vi "Main Editor UI.vi"() -> ()   [LabVIEW 2013, in "Shared Memory editor node.lvclass"]
doc: "This is the main view for configuration the behavior of a module in the DCAF standard editor."
uses:
  Shared Memory editor node.lvclass
  <vilib>/NI/Configuration Framework/Controls/EventCluster.ctl
  <vilib>/NI/Configuration Framework/NISE_CEF_TreeControl.lvlib
  <vilib>/NI/Configuration Framework/Node/UserEventRef.ctl
  <vilib>/NI/Configuration Framework/Node/NISE_CEF_Node.lvclass
  <vilib>/NI/Tools/Keyed Array/KeyedArray.ctl
  <vilib>/NI/Tools/Keyed Array/Tools_KeyedArray.lvlib
  <vilib>/NI/AMC/Message.ctl
  <vilib>/NI/AMC/AMC.lvlib
  <vilib>/NI/AMC/Message Queue.ctl
  <vilib>/NI/Tag Bus/tag/tag descriptor.lvclass
  <vilib>/NI/Tag Bus Module Framework/channel/TBM channel.lvclass
  <vilib>/NI/DCAF/Tag Editor Core/Table API/Available Tag Menu/channel action event.ctl
  <vilib>/NI/DCAF/Tag Editor Core/Table API/Table Manager.lvlib
  <vilib>/NI/Configuration Framework/Node/NodeRef.ctl
  <vilib>/NI/Configuration Framework/Node/NodeChangeEvent.ctl
  <vilib>/NI/Configuration Framework/Node/CacheState.ctl
  <vilib>/NI/Configuration Framework/Node/RefreshUIEvent.ctl
  <vilib>/NI/Configuration Framework/Node/StopEvent.ctl
  <vilib>/NI/DCAF/Tag Editor Core/Table API/Table Manager/references.ctl
  <vilib>/NI/DCAF/Tag Editor Core/Table API/Table Manager/Table Manager.lvclass
  <vilib>/NI/DCAF/Tag Editor Core/Table API/Listbox/Multi Column Listbox.lvclass
  <vilib>/Utility/miscctls.llb/LVPositionTypeDef.ctl
  <vilib>/NI/DCAF UI Toolkit/Controls/DCAF UI Elements.lvlib
  <vilib>/NI/DCAF/Tag Editor Core/Table API/Table Manager/Call Back Ref Type Def.ctl
  <vilib>/NI/DCAF/Tag Editor Core/Table API/Available Tag Menu/dialog output action.ctl
  <vilib>/NI/DCAF/Tag Editor Core/Configuration Editor/Classes/Engine Parent/Engine Parent Editor Node.lvclass
  <vilib>/NI/DCAF/Tag Editor Core/Configuration Editor/Classes/Module editor node/module editor node.lvclass
  module/configuration/Shared Memory configuration.lvclass
  <vilib>/NI/Tag Bus/tag/Data Type.ctl
  Permissions Enum.ctl
  sync/sync item.ctl
  sync/sync mechanism.ctl
  <vilib>/NI/DCAF UI Toolkit/Controls/Add.ctl
  <vilib>/NI/DCAF UI Toolkit/Controls/Remove.ctl
  <vilib>/NI/DCAF UI Toolkit/Controls/Configure.ctl
panel:
  in  "user event out":refnum<user-event>
  in  "Permissions":T1=enum."Read from Memory"
  in  "data type":T2
  in  "node change":T3
  in  "cache state":T4
  in  "refresh UI":T5
  in  "stop event":T6
  in  "Tab Control":T7(tab)
  in  "Remove Button":T8
  in  "Add Button":T9
  in  "Table":i32(listbox)
  in  "settings":T10
  in  "output file string":string caption="output file string (optional)"
  in  "input file string":string caption="input file string (optional)"
  in  "minor":dbl
  in  "major":dbl
  in  "C header":bool
  in  "c header file string":string caption="C header file string (optional)"
  in  "c header file directory":path caption="C header file directory"
  in  "Shared memory name":string="dcaf_sync"
  out "Struct prototype":string="struct dcaf_sync{\n   semt_t start_sem;\n};"
  in  "sync end of cycle":T11[](array[typedef])=[{"mechanism"=enum."Semaphore", "name"=""}]
  in  "sync start of cycle":T11[](array[typedef])
  in  "Struct name":string="dcaf_sync"
  in  "Timeout (us)":i32 step=25
  in  "Enable sync":bool
  in  "user event":T13
  in  "main queue":T14
  in  "node ref":T15
  # "Shared Memory Files (<EngineName>_<\"input/output\">_<DataType>_<FileString>)"
  # "The data file names will follow a fixed format with an optional appended user file name string. File input and output classification is from the perspective of an  external process (or application) which will access the file.\n\nExample: A C application running in parallel to the DCAF based LabVIEW Real-Time EXE application will view any file that it writes to as an \"output\" data file in Linux shared memory."
  # "C Header File Generation"
  # "Generate a C header file in a \"C header file directory\" which contains shared memory mapping information for use in C applications. The default C header file name will use the configuration file name and add optional user \"C header file string\" text: \n\n<ConfigurationFileName>_<FileString>.h\n\nThe user will override the file name format if the \".h\" file extension is included. The \"version\" will be added to the header file as a #define declaration in the header file."
  # "version"
  # "Start of cycle"
  # "End of cycle (optional response)"
  # "Mechanism"
  # "Name in struct"
  # "Mechanism"
  # "Name in struct"
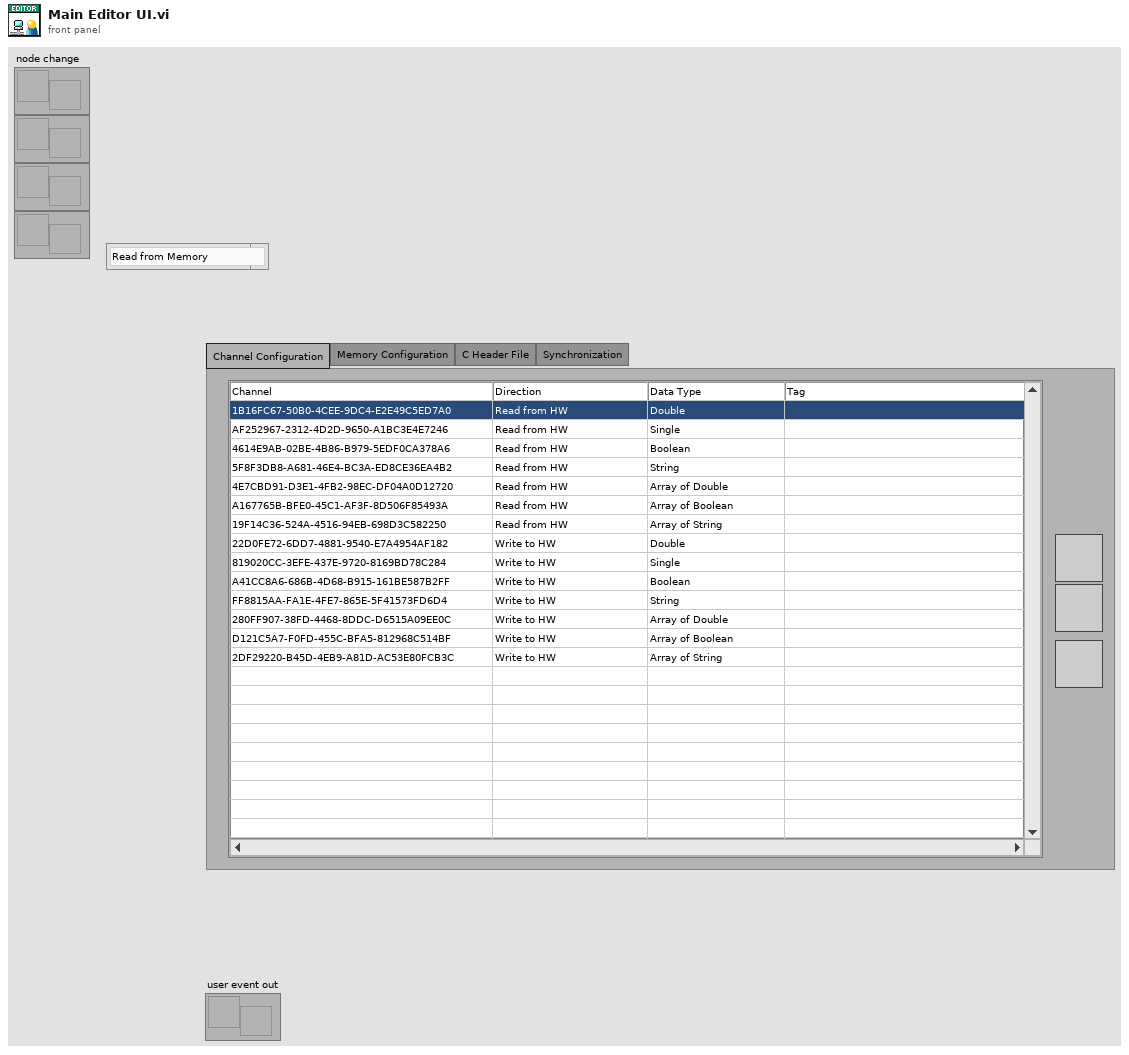
[diagram p1: front panel]
types:
  T1 = typedef "Shared Memory editor node.lvclass/Permissions Enum.ctl" = enum16{"Write to Memory", "Read from Memory"}
  T2 = typedef "tag bus.lvlib/tag descriptor.lvclass/Data Type.ctl" = enum16{"Double", "Single", "I64", "I32", "I16", "I8", "U64", "U32", "U16", "U8", "Boolean", "String", "Array of Double", "Array of Single", "Array of I64", "Array of I32", "Array of I16", "Array of I8", "Array of U64", "Array of U32", "Array of U16", "Array of U8", "Array of Boolean", "Array of String"}
  T3 = typedef "NISE_CEF_Node.lvclass/NodeChangeEvent.ctl" = refnum<user-event>
  T4 = typedef "NISE_CEF_Node.lvclass/CacheState.ctl" = refnum<user-event>
  T5 = typedef "NISE_CEF_Node.lvclass/RefreshUIEvent.ctl" = refnum<user-event>
  T6 = typedef "NISE_CEF_Node.lvclass/StopEvent.ctl" = refnum<user-event>
  T7 = enum32{"Channel Configuration", "Memory Configuration", "C Header File", "Synchronization"}
  T8 = typedef "DCAF UI Elements.lvlib/Remove.ctl" = bool
  T9 = typedef "DCAF UI Elements.lvlib/Add.ctl" = bool
  T10 = typedef "DCAF UI Elements.lvlib/Configure.ctl" = bool
  T11 = typedef "Shared Memory configuration.lvclass/sync item.ctl" = cluster{"mechanism":T12, "name":string}
  T12 = typedef "Shared Memory configuration.lvclass/sync mechanism.ctl" = enum16{"Semaphore", "Conditional Variable"}
  T13 = typedef "NISE_CEF_Node.lvclass/UserEventRef.ctl" = refnum<user-event>
  T14 = typedef "AMC.lvlib/Message Queue.ctl" = refnum<queue>
  T15 = typedef "NISE_CEF_Node.lvclass/NodeRef.ctl" = refnum<data-value>
  T16 = typedef "Table Manager.lvlib/Table Manager.lvclass/references.ctl" = cluster{"stop event":T6, "refresh UI":T5, "cache state":T4, "node change":T3, "user event out":refnum<user-event>, "main queue":T14, "user event":T13}
  T17 = typedef "LVPositionTypeDef.ctl" = cluster{"Left":i32, "Top":i32}
  T18 = typedef "Table Manager.lvlib/Table Manager.lvclass/object ref.ctl" = cluster{"engine":refnum<data-value>, "Node Ref":refnum<data-value>}
  T19 = typedef "Table Manager.lvlib/Column.lvclass/Column Descriptor.ctl" = cluster{"name":string, "caption":string, "Column Type":T20, "Params":string, "AutoSizeMode":i32, "FillWeight":sgl, "MinWidth":u32, "tooltip":string, "Enum Reference":refnum<vi>, "Channel suffix":string, "Read Only":bool, "Call Back VI":T21, "DT Dependency":i32, "name dependency":i32, "data type":T2, "Custom Column":refnum<class "Column.lvclass">}
  T20 = typedef "Table Manager.lvlib/Column.lvclass/Column Type.ctl" = enum16{"String", "Mapping", "Enum", "Custom"}
  T21 = typedef "Table Manager.lvlib/Table Manager.lvclass/Call Back Ref Type Def.ctl" = refnum<vi>
  T22 = typedef "Table Manager.lvlib/Table Manager.lvclass/Table Events.ctl" = cluster{"Menu Selection":refnum<user-event>}
  T23 = enum8{"Enabled", "Disabled", "Disabled and Grayed Out"}
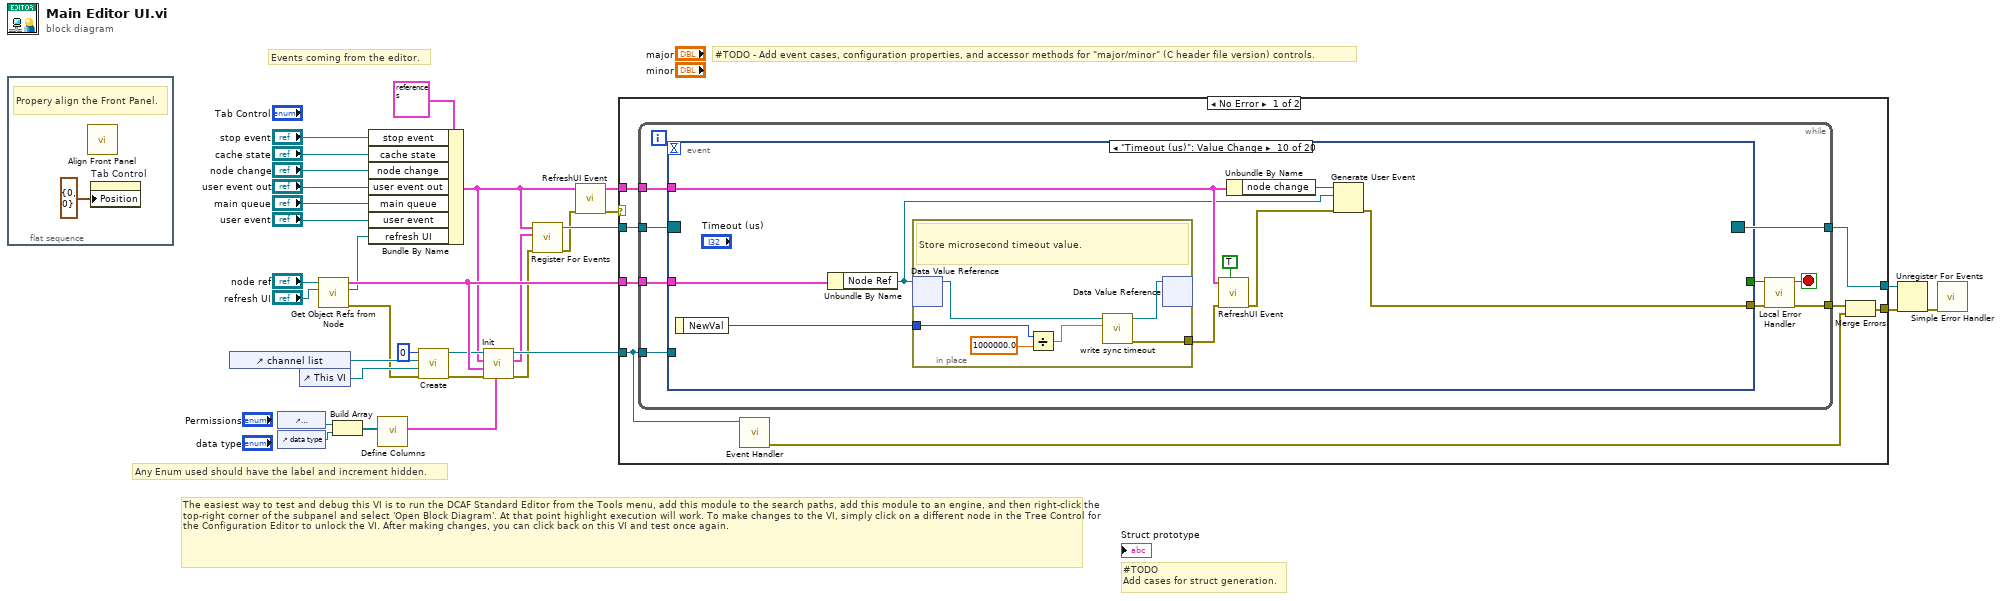
[diagram p0: block diagram]
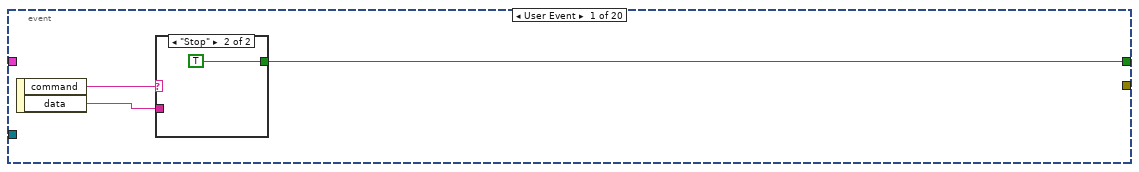
[diagram p2: hidden frame]
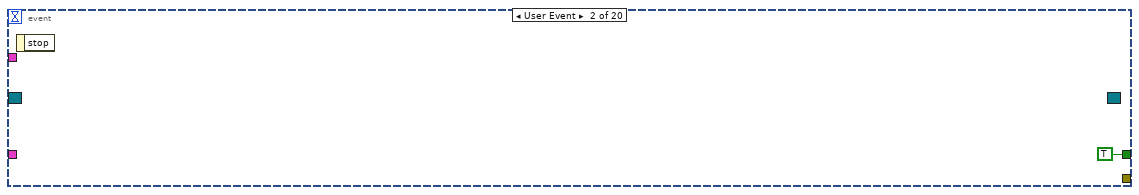
[diagram p4: hidden frame]
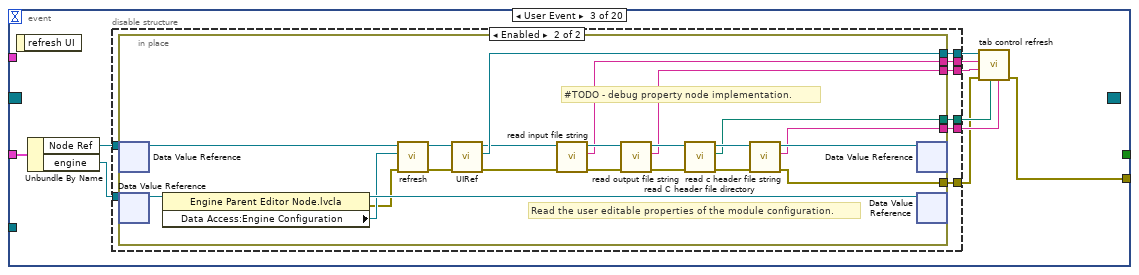
[diagram p5: hidden frame]
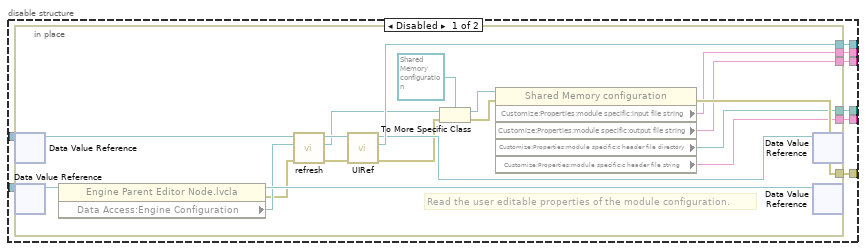
[diagram p6: hidden frame]
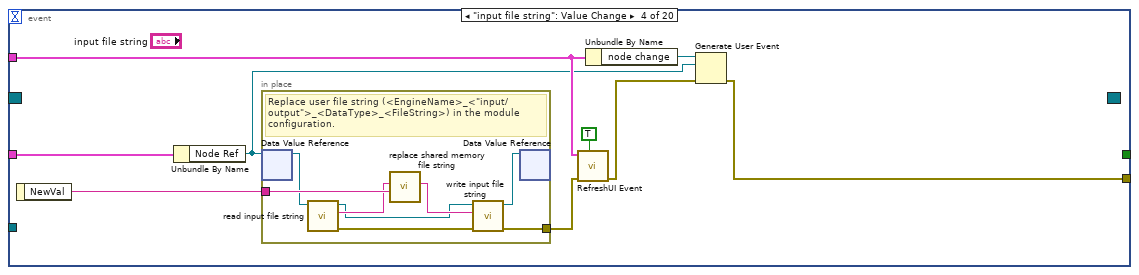
[diagram p7: hidden frame]
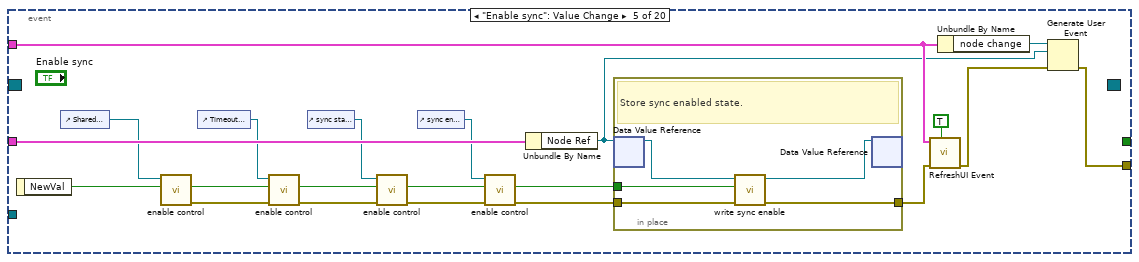
[diagram p8: hidden frame]
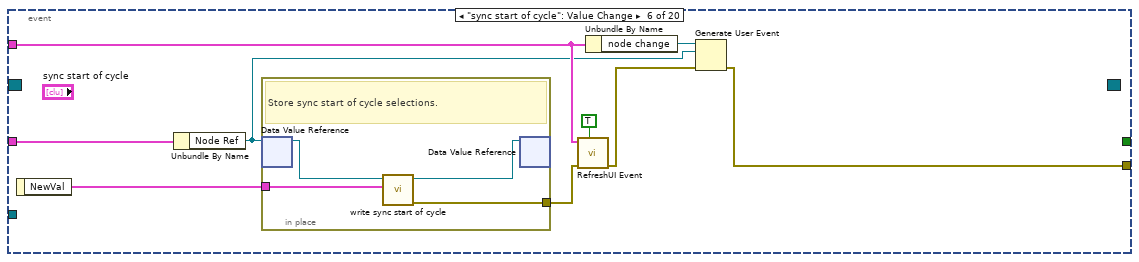
[diagram p9: hidden frame]
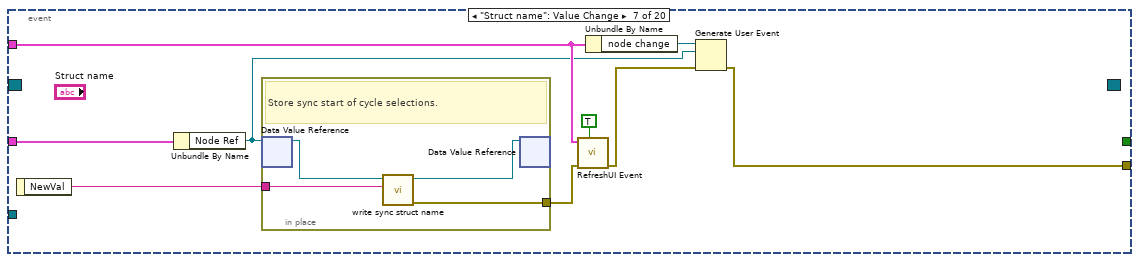
[diagram p10: hidden frame]
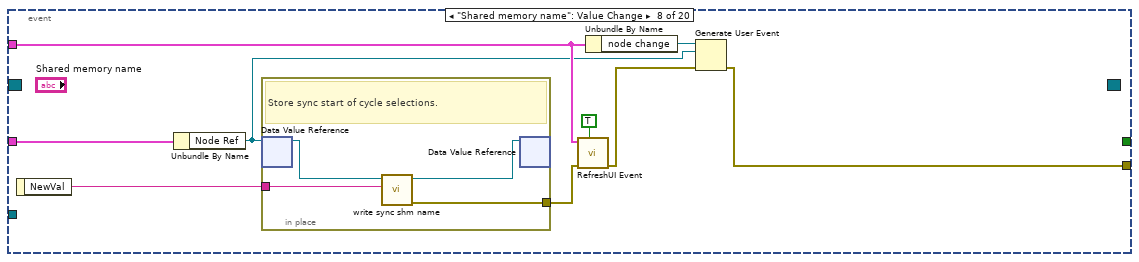
[diagram p11: hidden frame]
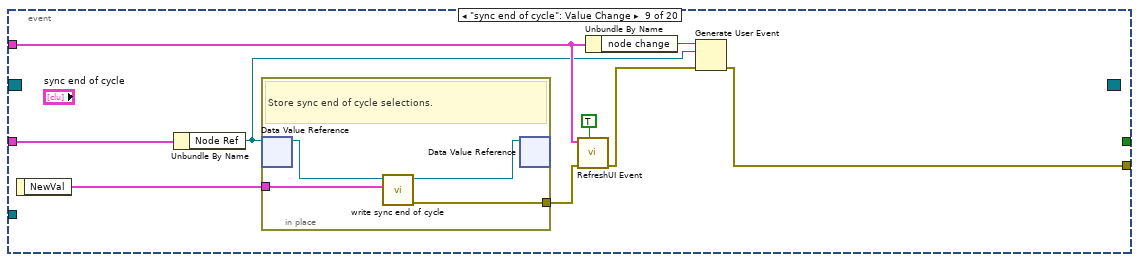
[diagram p12: hidden frame]
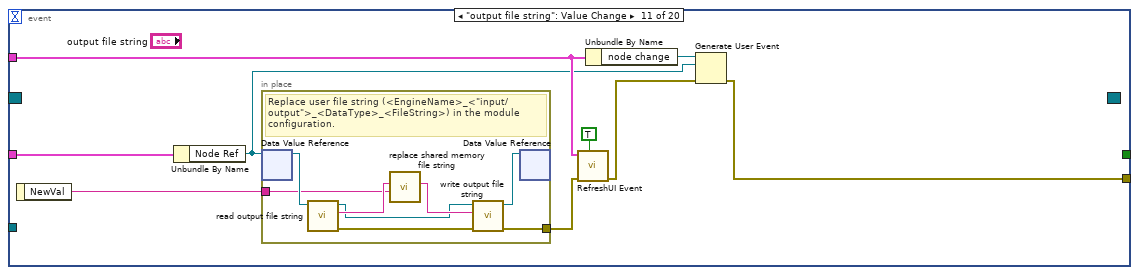
[diagram p13: hidden frame]
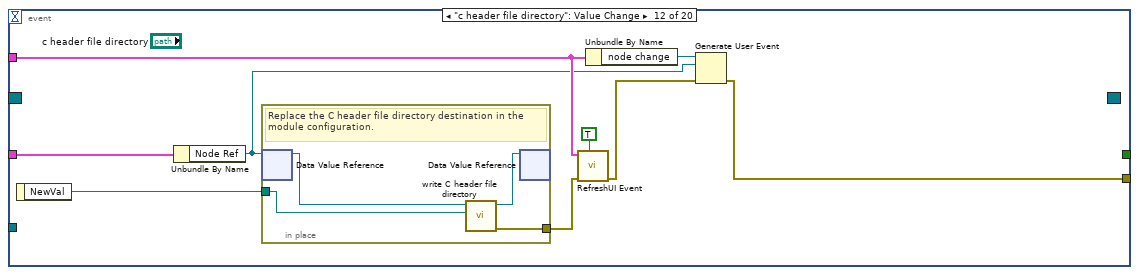
[diagram p14: hidden frame]
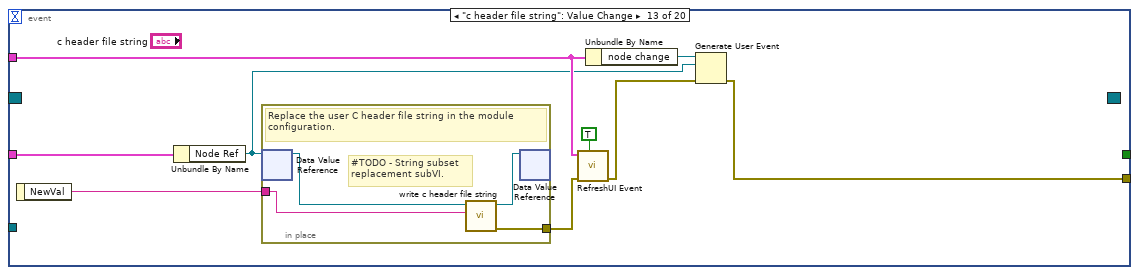
[diagram p15: hidden frame]
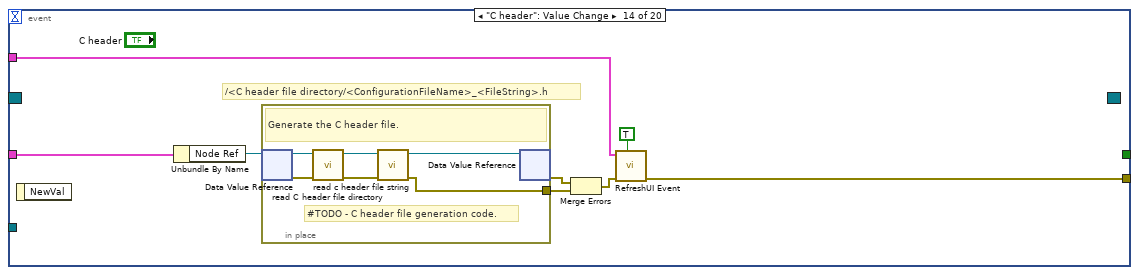
[diagram p16: hidden frame]
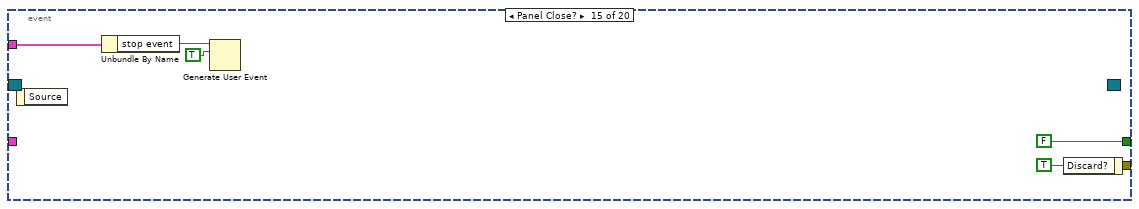
[diagram p17: hidden frame]
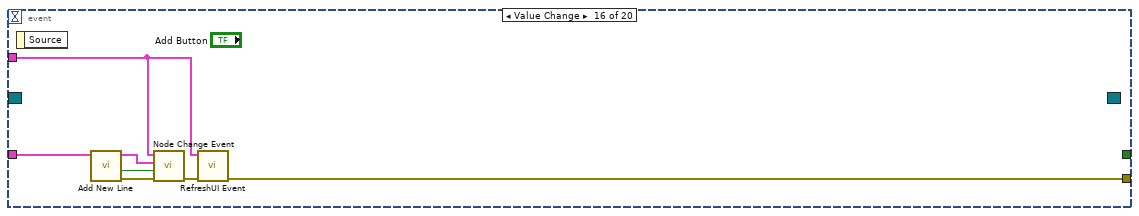
[diagram p18: hidden frame]
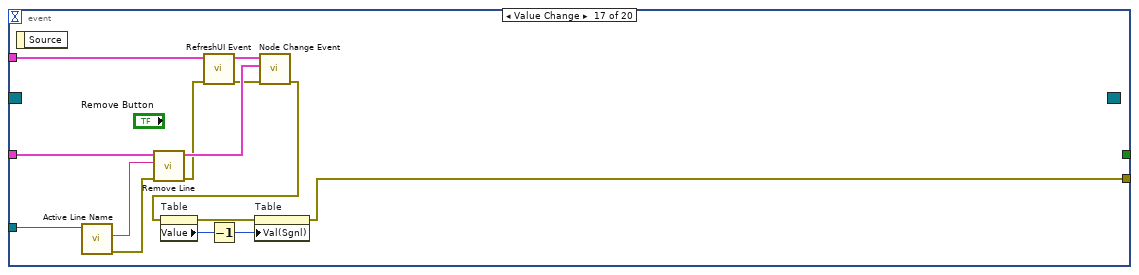
[diagram p19: hidden frame]
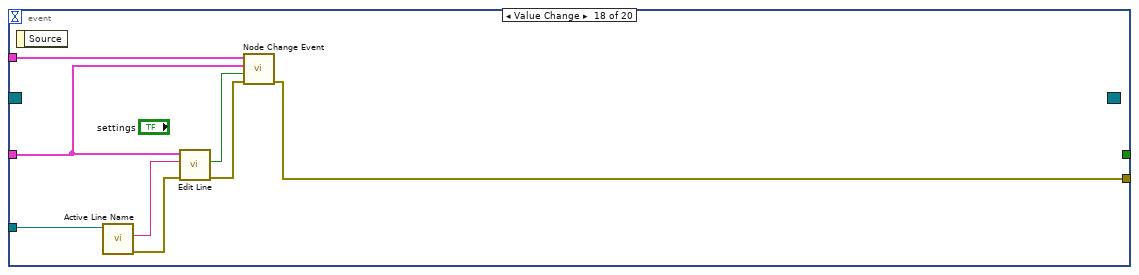
[diagram p20: hidden frame]
diagram:
  # "#TODO\nAdd cases for struct generation."
  # "#TODO - Add event cases, configuration properties, and accessor methods for \"major/minor\" (C header file version) controls."
  # "The easiest way to test and debug this VI is to run the DCAF Standard Editor from the Tools menu, add this module to the search paths, add this module to an engine, and then right-click the top-right corner of the subpanel and select 'Open Block Diagram'. At that point highlight execution will work. To make changes to the VI, simply click on a different node in the Tree Control for the Configuration Editor to unlock the VI. After making changes, you can click back on this VI and test once again."
  # "Any Enum used should have the label and increment hidden."
  # "Events coming from the editor."
  n1 = flat-sequence {
    frame #0 {
      # "Propery align the Front Panel."
      n2 = call <vilib>:"Align Front Panel.vi"() -> ()  [unwired: 10 in, 2 out]
      n3 = property on="Tab Control" class="TabCtl (strict)"("Position"=T17 {"Left"=0, "Top"=0}) -> ()  [unwired: 2 in, 2 out]
    }
  }
  n4 = control-ref of="channel list"() -> (w9:refnum<vi>)
  n5 = control-ref of="Permissions"() -> (w19:refnum<vi>)
  n6 = control-ref of="data type"() -> (w18:refnum<vi>)
  n7 = control-ref of="This VI"() -> (w7:refnum<vi>)
  n8 = call "Get Object Refs from Node.vi"("Refresh UI"="refresh UI", "Data Value Reference in"="node ref") -> ("error out"=w4:errorcluster, "Refresh UI out"=w2:T5, "References"=w16:T18)  [unwired: 7 in]
  n9 = Build Array(w19, w18) -> (w17:refnum<vi>[])
  n10 = Bundle By Name(cluster=T16 {"stop event"=refnum, "refresh UI"=refnum, "cache state"=refnum, "node change"=refnum, "user event out"=refnum, "main queue"=refnum, "user event"=refnum} ("References"), "stop event"="stop event", "cache state"="cache state", "node change"="node change", "user event out"="user event out", "main queue"="main queue", "user event"="user event", "refresh UI"=w2) -> (w1:T16)
  n11 = call "Define Columns.vi"("Enum Array"=w17) -> ("Column Definition"=w21:T19[])  [unwired: 10 in]
  n12 = call <vilib>:"Create.vi"("error in (no error)"=w4, "Top VI"=w7, "Listbox"=w9, "Index"=0) -> ("error out"=w5:errorcluster, "reference out"=w6:refnum<class "Multi Column Listbox.lvclass">)  [unwired: 6 in]
  n13 = call-dynamic "Init.vi"("Column Descriptors"=w21, "error in (no error)"=w5, "Node object refs"=w16, "Event References"=w1, "Multi Column Listbox in"=w6) -> ("error out"=w11:errorcluster, "Table Events"=w10:T22, "Multi Column Listbox out"=w15:refnum<class "Multi Column Listbox.lvclass">)  [unwired: 4 in]
  n14 = call "Register For Events.vi"("error in"=w11, "Table Events"=w10, "References"=w1) -> ("error out"=w13:errorcluster, "Event Registration Refnum"=w22:refnum<event-registration>)  [unwired: 7 in]
  n15 = call "RefreshUI Event.vi"("error in (no error)"=w13, "References in"=w1) -> ("error out"=w12:errorcluster, "References out"=w20:T16)  [unwired: 8 in]
  n16 = case shown="No Error" w12 {
    selector: w12 -> [_ w346]
    tunnel: w22 -> [w41 w345]
    tunnel: [w40 w345] -> w32
    tunnel: [w34 w346] -> w31
    tunnel: w20 -> [w39 _]
    tunnel: w16 -> [w38 _]
    tunnel: w15 -> [w37 _]
    frame No Error {
      n17 = while {
        tunnel: w41 -> [w50]
        tunnel: [w49] -> w40
        tunnel: [w46] -> w35
        tunnel: w39 -> [w44]
        tunnel: w38 -> [w43]
        tunnel: w37 -> [w42]
        stop <- w48 stop-if-true
        n18 = event shown="[9] \"Timeout (us)\": Value Change" {
          selector: w50 -> [_ _ _ _ _ _ _ _ _ _ _ _ _ _ _ _ _ _ _ _]
          dyn-events: [_ _ _ _ _ _ _ _ _ _ _ _ _ _ _ _ _ _ _ _] -> w49
          timeout: _ -> [_ _ _ _ _ _ _ _ _ _ _ _ _ _ _ _ _ _ _ _]
          tunnel: [w53 TRUE _ _ _ _ _ _ _ _ _ _ _ _ FALSE _ _ _ _ _] -> w47
          tunnel: [_ _ w56 w123 w154 w166 w179 w192 w205 w218 w234 w251 w265 w276 _ w295 w302 w319 w327 _] -> w45
          tunnel: w44 -> [_ _ _ w127 w158 w170 w183 w196 w209 w222 w236 w253 w266 w278 w291 w299 w313 w321 w323 _]
          tunnel: w43 -> [_ _ w57 w129 w159 w172 w185 w198 w211 w224 w239 w256 w269 w283 _ w300 w312 w317 w324 _]
          tunnel: w42 -> [_ _ _ _ _ _ _ _ _ _ _ _ _ _ _ _ w308 w318 _ _]
          event User Event {
            n19 = event-data() -> ("command"=w52:string, "data"=w51:string)  [unwired: 1 in]
            n20 = case shown="\"Stop\"" w52 {
              tunnel: [_ TRUE] -> w53
              tunnel: w51 -> [_ _]
              frame Default {
              }
              frame "Stop" {
              }
            }
          }
          event User Event {
            n21 = event-data() -> ()  [unwired: 1 in, 1 out]
          }
          event User Event {
            n22 = event-data() -> ()  [unwired: 1 in, 1 out]
            n23 = Unbundle By Name(w57) -> ("Node Ref"=w58:refnum<data-value>, "engine"=w59:refnum<data-value>)
            n24 = disable-structure shown="Enabled" {
              disable-tunnel: [w73 w100] -> w65
              disable-tunnel: [w72 w93] -> w64
              disable-tunnel: [w71 w94] -> w63
              disable-tunnel: [w70 w95] -> w62
              disable-tunnel: [w69 w96] -> w61
              disable-tunnel: [w68 w97] -> w60
              disable-tunnel: w59 -> [w67 w99]
              disable-tunnel: w58 -> [w66 w98]
              frame Disabled {
                n25 = in-place {
                  in-place-border: [w91] -> w68
                  in-place-border: [w90] -> w73
                  in-place-border: [w89] -> w69
                  in-place-border: [w88] -> w70
                  in-place-border: [w87] -> w71
                  in-place-border: [w86] -> w72
                  # "Read the user editable properties of the module configuration."
                  n26 = in-place-dvr #1(w66) -> (w83:refnum<class "module editor node.lvclass">)  [unwired: 1 out]
                  n27 = in-place-dvr #2(w67) -> (w92:refnum<class "Engine Parent Editor Node.lvclass">)  [unwired: 1 out]
                  n28 = property class="Engine Parent Editor Node.lvcla"(reference=w92) -> (reference out=w84:refnum<class "Engine Parent Editor Node.lvclass">, error out=w80:errorcluster, "Data Access:Engine Configuration"=w81:refnum<class "engine configuration.lvclass">)  [unwired: 1 in]
                  n29 = call-dynamic "refresh.vi"("error in (no error)"=w80, "Engine Configuration In"=w81, "Module Editor Node In"=w83) -> ("error out"=w79:errorcluster, "Engine Configuration Out"=w75:refnum<class "engine configuration.lvclass">, "Module Editor Node Out"=w82:refnum<class "module editor node.lvclass">)  [unwired: 6 in]
                  n30 = call-dynamic "UIRef.vi"("error in"=w79, "node in"=w82) -> ("error out"=w74:errorcluster, "VI refnum"=w90:refnum<vi>, "node out"=w85:refnum<class "module editor node.lvclass">)  [unwired: 7 in]
                  n31 = To More Specific Class(target class=refnum<class "Shared Memory configuration.lvclass"> refnum ("shared memory configuration"), reference=w75, error in=w74) -> (specific class reference=w77:refnum<class "Shared Memory configuration.lvclass">, error out=w76:errorcluster)
                  n32 = property class="Shared Memory configuration"(reference=w77, error in=w76) -> (error out=w91:errorcluster, "Customize:Properties:module specific:input file string"=w89:string, "Customize:Properties:module specific:output file string"=w88:string, "Customize:Properties:module specific:c header file directory"=w87:path, "Customize:Properties:module specific:c header file string"=w86:string)  [unwired: 1 out]
                  n33 = in-place-dvr #1(w85) -> ()  [unwired: 2 out]
                  n34 = in-place-dvr #2(w84) -> ()  [unwired: 2 out]
                }
              }
              frame Enabled {
                n35 = in-place {
                  in-place-border: [w121] -> w100
                  in-place-border: [w105] -> w97
                  in-place-border: [w104] -> w96
                  in-place-border: [w103] -> w95
                  in-place-border: [w102] -> w94
                  in-place-border: [w101] -> w93
                  # "#TODO - debug property node implementation."
                  # "Read the user editable properties of the module configuration."
                  n36 = in-place-dvr #3(w98) -> (w119:refnum<class "module editor node.lvclass">)  [unwired: 1 out]
                  n37 = in-place-dvr #4(w99) -> (w122:refnum<class "Engine Parent Editor Node.lvclass">)  [unwired: 1 out]
                  n38 = property class="Engine Parent Editor Node.lvcla"(reference=w122) -> (reference out=w120:refnum<class "Engine Parent Editor Node.lvclass">, error out=w116:errorcluster, "Data Access:Engine Configuration"=w117:refnum<class "engine configuration.lvclass">)  [unwired: 1 in]
                  n39 = call-dynamic "refresh.vi"("error in (no error)"=w116, "Engine Configuration In"=w117, "Module Editor Node In"=w119) -> ("error out"=w115:errorcluster, "Module Editor Node Out"=w118:refnum<class "module editor node.lvclass">)  [unwired: 6 in, 1 out]
                  n40 = call-dynamic "UIRef.vi"("error in"=w115, "node in"=w118) -> ("error out"=w109:errorcluster, "VI refnum"=w121:refnum<vi>, "node out"=w111:refnum<class "module editor node.lvclass">)  [unwired: 7 in]
                  n41 = call "read input file string.vi"("error in"=w109, "shared memory editor node"=w111) -> ("error out"=w108:errorcluster, "input file string"=w104:string, "shared memory editor node out"=w114:refnum<class "module editor node.lvclass">)  [unwired: 7 in]
                  n42 = call "read output file string.vi"("error in"=w108, "shared memory editor node"=w114) -> ("error out"=w107:errorcluster, "output file string"=w103:string, "shared memory editor node out"=w113:refnum<class "module editor node.lvclass">)  [unwired: 7 in]
                  n43 = call "read C header file directory.vi"("error in"=w107, "shared memory editor node"=w113) -> ("error out"=w106:errorcluster, "C header file directory"=w102:path, "shared memory editor node out"=w112:refnum<class "module editor node.lvclass">)  [unwired: 7 in]
                  n44 = call "read c header file string.vi"("error in"=w106, "shared memory editor node"=w112) -> ("error out"=w105:errorcluster, "c header file string"=w101:string, "shared memory editor node out"=w110:refnum<class "module editor node.lvclass">)  [unwired: 7 in]
                  n45 = in-place-dvr #3(w110) -> ()  [unwired: 2 out]
                  n46 = in-place-dvr #4(w120) -> ()  [unwired: 2 out]
                }
              }
            }
            n47 = call "tab control refresh.vi"("c header file string"=w64, "C header file directory"=w63, "error in"=w60, "output file string"=w62, "input file string"=w61, "VI reference"=w65) -> ("error out"=w56:errorcluster)  [unwired: 5 in]
          }
          event "input file string": Value Change {
            n48 = event-data() -> ("NewVal"=w128:string)  [unwired: 1 in]
            n49 = Unbundle By Name(w129) -> ("Node Ref"=w125:refnum<data-value>)
            n50 = in-place {
              in-place-border: w128 -> [w136]
              in-place-border: [w137] -> w131
              # "Replace user file string (<EngineName>_<\"input/output\">_<DataType>_<FileString>) in the module configuration."
              n51 = in-place-dvr #5(w125) -> (w134:refnum<class "module editor node.lvclass">)  [unwired: 1 out]
              n52 = call "read input file string.vi"("shared memory editor node"=w134) -> ("error out"=w138:errorcluster, "input file string"=w135:string, "shared memory editor node out"=w132:refnum<class "module editor node.lvclass">)  [unwired: 8 in]
              n53 = call "replace shared memory file string.vi"("new string"=w136, "file name"=w135) -> ("new file name"=w133:string)  [unwired: 9 in]
              n54 = call "write input file string.vi"("error in"=w138, "input file string"=w133, "shared memory editor node"=w132) -> ("error out"=w137:errorcluster, "shared memory editor node out"=w139:refnum<class "module editor node.lvclass">)  [unwired: 7 in]
              n55 = in-place-dvr #5(w139) -> ()  [unwired: 2 out]
            }
            n56 = call "RefreshUI Event.vi"("Refresh (T)"=TRUE, "error in (no error)"=w131, "References in"=w127) -> ("error out"=w124:errorcluster)  [unwired: 7 in, 1 out]
            n57 = Unbundle By Name(w127) -> ("node change"=w126:T3)
            n58 = Generate User Event(user event=w126, event data cluster=w125, error in=w124) -> (error out=w123:errorcluster)  [unwired: 1 in, 1 out]
          }
          event "Enable sync": Value Change {
            n59 = event-data() -> ("NewVal"=w142:bool)  [unwired: 1 in]
            n60 = control-ref of="Shared memory name"() -> (w140:refnum<vi>)
            n61 = call "enable control.vi"("enabled? (T)"=w142, "control in"=w140) -> ("error out"=w143:errorcluster, "enabled out"=w141:bool)  [unwired: 7 in, 1 out]
            n62 = control-ref of="Timeout (us)"() -> (w146:refnum<vi>)
            n63 = call "enable control.vi"("error in (no error)"=w143, "enabled? (T)"=w141, "control in"=w146) -> ("error out"=w152:errorcluster, "enabled out"=w149:bool)  [unwired: 6 in, 1 out]
            n64 = control-ref of="sync start of cycle"() -> (w145:refnum<vi>)
            n65 = call "enable control.vi"("error in (no error)"=w152, "enabled? (T)"=w149, "control in"=w145) -> ("error out"=w151:errorcluster, "enabled out"=w148:bool)  [unwired: 6 in, 1 out]
            n66 = control-ref of="sync end of cycle"() -> (w144:refnum<vi>)
            n67 = call "enable control.vi"("error in (no error)"=w151, "enabled? (T)"=w148, "control in"=w144) -> ("error out"=w150:errorcluster, "enabled out"=w147:bool)  [unwired: 6 in, 1 out]
            n68 = Unbundle By Name(w159) -> ("Node Ref"=w156:refnum<data-value>)
            n69 = in-place {
              in-place-border: w147 -> [w162]
              in-place-border: [w165] -> w153
              in-place-border: w150 -> [w161]
              # "Store sync enabled state."
              n70 = in-place-dvr #6(w156) -> (w164:refnum<class "module editor node.lvclass">)  [unwired: 1 out]
              n71 = call "write sync enable.vi"("error in"=w161, "sync enable"=w162, "shared memory editor node"=w164) -> ("error out"=w165:errorcluster, "shared memory editor node out"=w163:refnum<class "module editor node.lvclass">)  [unwired: 7 in]
              n72 = in-place-dvr #6(w163) -> ()  [unwired: 2 out]
            }
            n73 = call "RefreshUI Event.vi"("Refresh (T)"=TRUE, "error in (no error)"=w153, "References in"=w158) -> ("error out"=w155:errorcluster)  [unwired: 7 in, 1 out]
            n74 = Unbundle By Name(w158) -> ("node change"=w157:T3)
            n75 = Generate User Event(user event=w157, event data cluster=w156, error in=w155) -> (error out=w154:errorcluster)  [unwired: 1 in, 1 out]
          }
          event "sync start of cycle": Value Change {
            n76 = event-data() -> ("NewVal"=w171:T11[])  [unwired: 1 in]
            n77 = Unbundle By Name(w172) -> ("Node Ref"=w168:refnum<data-value>)
            n78 = in-place {
              in-place-border: w171 -> [w175]
              in-place-border: [w178] -> w174
              # "Store sync start of cycle selections."
              n79 = in-place-dvr #7(w168) -> (w176:refnum<class "module editor node.lvclass">)  [unwired: 1 out]
              n80 = call "write sync start of cycle.vi"("sync start of cycle"=w175, "shared memory editor node"=w176) -> ("error out"=w178:errorcluster, "shared memory editor node out"=w177:refnum<class "module editor node.lvclass">)  [unwired: 8 in]
              n81 = in-place-dvr #7(w177) -> ()  [unwired: 2 out]
            }
            n82 = call "RefreshUI Event.vi"("Refresh (T)"=TRUE, "error in (no error)"=w174, "References in"=w170) -> ("error out"=w167:errorcluster)  [unwired: 7 in, 1 out]
            n83 = Unbundle By Name(w170) -> ("node change"=w169:T3)
            n84 = Generate User Event(user event=w169, event data cluster=w168, error in=w167) -> (error out=w166:errorcluster)  [unwired: 1 in, 1 out]
          }
          event "Struct name": Value Change {
            n85 = event-data() -> ("NewVal"=w184:string)  [unwired: 1 in]
            n86 = Unbundle By Name(w185) -> ("Node Ref"=w181:refnum<data-value>)
            n87 = in-place {
              in-place-border: w184 -> [w188]
              in-place-border: [w191] -> w187
              # "Store sync start of cycle selections."
              n88 = in-place-dvr #8(w181) -> (w189:refnum<class "module editor node.lvclass">)  [unwired: 1 out]
              n89 = call "write sync struct name.vi"("struct name"=w188, "shared memory editor node"=w189) -> ("error out"=w191:errorcluster, "shared memory editor node out"=w190:refnum<class "module editor node.lvclass">)  [unwired: 8 in]
              n90 = in-place-dvr #8(w190) -> ()  [unwired: 2 out]
            }
            n91 = call "RefreshUI Event.vi"("Refresh (T)"=TRUE, "error in (no error)"=w187, "References in"=w183) -> ("error out"=w180:errorcluster)  [unwired: 7 in, 1 out]
            n92 = Unbundle By Name(w183) -> ("node change"=w182:T3)
            n93 = Generate User Event(user event=w182, event data cluster=w181, error in=w180) -> (error out=w179:errorcluster)  [unwired: 1 in, 1 out]
          }
          event "Shared memory name": Value Change {
            n94 = event-data() -> ("NewVal"=w197:string)  [unwired: 1 in]
            n95 = Unbundle By Name(w198) -> ("Node Ref"=w194:refnum<data-value>)
            n96 = in-place {
              in-place-border: w197 -> [w201]
              in-place-border: [w204] -> w200
              # "Store sync start of cycle selections."
              n97 = in-place-dvr #9(w194) -> (w202:refnum<class "module editor node.lvclass">)  [unwired: 1 out]
              n98 = call "write sync shm name.vi"("shm name"=w201, "shared memory editor node"=w202) -> ("error out"=w204:errorcluster, "shared memory editor node out"=w203:refnum<class "module editor node.lvclass">)  [unwired: 8 in]
              n99 = in-place-dvr #9(w203) -> ()  [unwired: 2 out]
            }
            n100 = call "RefreshUI Event.vi"("Refresh (T)"=TRUE, "error in (no error)"=w200, "References in"=w196) -> ("error out"=w193:errorcluster)  [unwired: 7 in, 1 out]
            n101 = Unbundle By Name(w196) -> ("node change"=w195:T3)
            n102 = Generate User Event(user event=w195, event data cluster=w194, error in=w193) -> (error out=w192:errorcluster)  [unwired: 1 in, 1 out]
          }
          event "sync end of cycle": Value Change {
            n103 = event-data() -> ("NewVal"=w210:T11[])  [unwired: 1 in]
            n104 = Unbundle By Name(w211) -> ("Node Ref"=w207:refnum<data-value>)
            n105 = in-place {
              in-place-border: w210 -> [w214]
              in-place-border: [w217] -> w213
              # "Store sync end of cycle selections."
              n106 = in-place-dvr #10(w207) -> (w215:refnum<class "module editor node.lvclass">)  [unwired: 1 out]
              n107 = call "write sync end of cycle.vi"("sync end of cycle"=w214, "shared memory editor node"=w215) -> ("error out"=w217:errorcluster, "shared memory editor node out"=w216:refnum<class "module editor node.lvclass">)  [unwired: 8 in]
              n108 = in-place-dvr #10(w216) -> ()  [unwired: 2 out]
            }
            n109 = call "RefreshUI Event.vi"("Refresh (T)"=TRUE, "error in (no error)"=w213, "References in"=w209) -> ("error out"=w206:errorcluster)  [unwired: 7 in, 1 out]
            n110 = Unbundle By Name(w209) -> ("node change"=w208:T3)
            n111 = Generate User Event(user event=w208, event data cluster=w207, error in=w206) -> (error out=w205:errorcluster)  [unwired: 1 in, 1 out]
          }
          event "Timeout (us)": Value Change {
            n112 = event-data() -> ("NewVal"=w223:i32)  [unwired: 1 in]
            n113 = Unbundle By Name(w224) -> ("Node Ref"=w220:refnum<data-value>)
            n114 = in-place {
              in-place-border: w223 -> [w228]
              in-place-border: [w232] -> w226
              # "Store microsecond timeout value."
              n115 = in-place-dvr #11(w220) -> (w230:refnum<class "module editor node.lvclass">)  [unwired: 1 out]
              n116 = Divide(x=w228, y=1000000.0) -> (x/y=w227:dbl)
              n117 = call "write sync timeout.vi"("sync timeout"=w227, "shared memory editor node"=w230) -> ("error out"=w232:errorcluster, "shared memory editor node out"=w231:refnum<class "module editor node.lvclass">)  [unwired: 8 in]
              n118 = in-place-dvr #11(w231) -> ()  [unwired: 2 out]
            }
            n119 = call "RefreshUI Event.vi"("Refresh (T)"=TRUE, "error in (no error)"=w226, "References in"=w222) -> ("error out"=w219:errorcluster)  [unwired: 7 in, 1 out]
            n120 = Unbundle By Name(w222) -> ("node change"=w221:T3)
            n121 = Generate User Event(user event=w221, event data cluster=w220, error in=w219) -> (error out=w218:errorcluster)  [unwired: 1 in, 1 out]
          }
          event "output file string": Value Change {
            n122 = event-data() -> ("NewVal"=w238:string)  [unwired: 1 in]
            n123 = Unbundle By Name(w239) -> ("Node Ref"=w235:refnum<data-value>)
            n124 = in-place {
              in-place-border: w238 -> [w244]
              in-place-border: [w246] -> w241
              # "Replace user file string (<EngineName>_<\"input/output\">_<DataType>_<FileString>) in the module configuration."
              n125 = in-place-dvr #12(w235) -> (w248:refnum<class "module editor node.lvclass">)  [unwired: 1 out]
              n126 = call "read output file string.vi"("shared memory editor node"=w248) -> ("error out"=w247:errorcluster, "output file string"=w245:string, "shared memory editor node out"=w242:refnum<class "module editor node.lvclass">)  [unwired: 8 in]
              n127 = call "replace shared memory file string.vi"("new string"=w244, "file name"=w245) -> ("new file name"=w243:string)  [unwired: 9 in]
              n128 = call "write output file string.vi"("error in"=w247, "output file string"=w243, "shared memory editor node"=w242) -> ("error out"=w246:errorcluster, "shared memory editor node out"=w249:refnum<class "module editor node.lvclass">)  [unwired: 7 in]
              n129 = in-place-dvr #12(w249) -> ()  [unwired: 2 out]
            }
            n130 = call "RefreshUI Event.vi"("Refresh (T)"=TRUE, "error in (no error)"=w241, "References in"=w236) -> ("error out"=w233:errorcluster)  [unwired: 7 in, 1 out]
            n131 = Unbundle By Name(w236) -> ("node change"=w237:T3)
            n132 = Generate User Event(user event=w237, event data cluster=w235, error in=w233) -> (error out=w234:errorcluster)  [unwired: 1 in, 1 out]
          }
          event "c header file directory": Value Change {
            n133 = event-data() -> ("NewVal"=w255:path)  [unwired: 1 in]
            n134 = Unbundle By Name(w256) -> ("Node Ref"=w250:refnum<data-value>)
            n135 = in-place {
              in-place-border: w255 -> [w259]
              in-place-border: [w261] -> w257
              # "Replace the C header file directory destination in the module configuration."
              n136 = in-place-dvr #13(w250) -> (w260:refnum<class "module editor node.lvclass">)  [unwired: 1 out]
              n137 = call "write C header file directory.vi"("C header file directory"=w259, "shared memory editor node"=w260) -> ("error out"=w261:errorcluster, "shared memory editor node out"=w262:refnum<class "module editor node.lvclass">)  [unwired: 8 in]
              n138 = in-place-dvr #13(w262) -> ()  [unwired: 2 out]
            }
            n139 = call "RefreshUI Event.vi"("Refresh (T)"=TRUE, "error in (no error)"=w257, "References in"=w253) -> ("error out"=w252:errorcluster)  [unwired: 7 in, 1 out]
            n140 = Unbundle By Name(w253) -> ("node change"=w254:T3)
            n141 = Generate User Event(user event=w254, event data cluster=w250, error in=w252) -> (error out=w251:errorcluster)  [unwired: 1 in, 1 out]
          }
          event "c header file string": Value Change {
            n142 = event-data() -> ("NewVal"=w268:string)  [unwired: 1 in]
            n143 = Unbundle By Name(w269) -> ("Node Ref"=w263:refnum<data-value>)
            n144 = in-place {
              in-place-border: w268 -> [w272]
              in-place-border: [w274] -> w270
              # "#TODO - String subset\nreplacement subVI."
              # "Replace the user C header file string in the module configuration."
              n145 = in-place-dvr #14(w263) -> (w273:refnum<class "module editor node.lvclass">)  [unwired: 1 out]
              n146 = call "write c header file string.vi"("c header file string"=w272, "shared memory editor node"=w273) -> ("error out"=w274:errorcluster, "shared memory editor node out"=w275:refnum<class "module editor node.lvclass">)  [unwired: 8 in]
              n147 = in-place-dvr #14(w275) -> ()  [unwired: 2 out]
            }
            n148 = call "RefreshUI Event.vi"("Refresh (T)"=TRUE, "error in (no error)"=w270, "References in"=w266) -> ("error out"=w264:errorcluster)  [unwired: 7 in, 1 out]
            n149 = Unbundle By Name(w266) -> ("node change"=w267:T3)
            n150 = Generate User Event(user event=w267, event data cluster=w263, error in=w264) -> (error out=w265:errorcluster)  [unwired: 1 in, 1 out]
          }
          event "C header": Value Change {
            # "/<C header file directory/<ConfigurationFileName>_<FileString>.h"
            n151 = event-data() -> ()  [unwired: 1 in, 1 out]
            n152 = Unbundle By Name(w283) -> ("Node Ref"=w282:refnum<data-value>)
            n153 = in-place {
              in-place-border: [w285] -> w280
              # "#TODO - C header file generation code."
              # "Generate the C header file."
              n154 = in-place-dvr #15(w282) -> (w288:refnum<class "module editor node.lvclass">, w284:errorcluster)
              n155 = call "read C header file directory.vi"("error in"=w284, "shared memory editor node"=w288) -> ("error out"=w289:errorcluster, "shared memory editor node out"=w287:refnum<class "module editor node.lvclass">)  [unwired: 7 in, 1 out]
              n156 = call "read c header file string.vi"("error in"=w289, "shared memory editor node"=w287) -> ("error out"=w285:errorcluster, "shared memory editor node out"=w286:refnum<class "module editor node.lvclass">)  [unwired: 7 in, 1 out]
              n157 = in-place-dvr #15(w286) -> (w281:errorcluster)  [unwired: 1 out]
            }
            n158 = Merge Errors(w281, w280) -> (w277:errorcluster)
            n159 = call "RefreshUI Event.vi"("Refresh (T)"=TRUE, "error in (no error)"=w277, "References in"=w278) -> ("error out"=w276:errorcluster)  [unwired: 7 in, 1 out]
          }
          event Panel Close? {
            n160 = event-data() -> ()  [unwired: 1 in, 1 out]
            n161 = Unbundle By Name(w291) -> ("stop event"=w290:T6)
            n162 = Generate User Event(user event=w290, event data cluster=TRUE ("event data")) -> ()  [unwired: 2 in, 2 out]
            n163 = event-data("Discard?"=TRUE) -> ()  [unwired: 1 in, 1 out]
          }
          event Value Change {
            n164 = event-data() -> ()  [unwired: 1 in, 1 out]
            n165 = call "Add New Line.vi"("objects"=w300) -> ("error out"=w298:errorcluster, "success"=w296:bool)  [unwired: 8 in, 1 out]
            n166 = call "Node Change Event.vi"("error in (no error)"=w298, "Send (T)"=w296, "objects"=w300, "References in"=w299) -> ("error out"=w297:errorcluster)  [unwired: 7 in]
            n167 = call "RefreshUI Event.vi"("error in (no error)"=w297, "References in"=w299) -> ("error out"=w295:errorcluster)  [unwired: 8 in, 1 out]
          }
          event Value Change {
            n168 = event-data() -> ()  [unwired: 1 in, 1 out]
            n169 = call-dynamic "Active Line Name.vi"("Multi Column Listbox in"=w308) -> ("error out"=w306:errorcluster, "Active Line Name"=w307:string)  [unwired: 8 in, 1 out]
            n170 = call "Remove Line.vi"("error in"=w306, "Active Line Name"=w307, "Objects"=w312) -> ("error out"=w309:errorcluster)  [unwired: 8 in]
            n171 = call "RefreshUI Event.vi"("error in (no error)"=w309, "References in"=w313) -> ("error out"=w311:errorcluster, "References out"=w310:T16)  [unwired: 8 in]
            n172 = call "Node Change Event.vi"("error in (no error)"=w311, "objects"=w312, "References in"=w310) -> ("error out"=w303:errorcluster)  [unwired: 8 in]
            n173 = property on="Table" class="MCListbox (strict)"(error in=w303) -> (error out=w301:errorcluster, "Value"=w304:i32)  [unwired: 1 in, 1 out]
            n174 = Decrement(x=w304) -> (x-1=w305:i32)
            n175 = property on="Table" class="MCListbox (strict)"(error in=w301, "Val(Sgnl)"=w305) -> (error out=w302:errorcluster)  [unwired: 1 in, 1 out]
          }
          event Value Change {
            n176 = event-data() -> ()  [unwired: 1 in, 1 out]
            n177 = call-dynamic "Active Line Name.vi"("Multi Column Listbox in"=w318) -> ("error out"=w315:errorcluster, "Active Line Name"=w316:string)  [unwired: 8 in, 1 out]
            n178 = call "Edit Line.vi"("error in"=w315, "Line Name"=w316, "References"=w317) -> ("error out"=w320:errorcluster, "change?"=w314:bool)  [unwired: 7 in]
            n179 = call "Node Change Event.vi"("error in (no error)"=w320, "Send (T)"=w314, "objects"=w317, "References in"=w321) -> ("error out"=w319:errorcluster)  [unwired: 7 in]
          }
          event User Event {
            n180 = event-data() -> ("Selected Value"=w329:string, "Line Name"=w326:string)  [unwired: 1 in]
            n181 = case shown="\"Add\"" w329 {
              tunnel: w326 -> [w332 _ w338]
              tunnel: w324 -> [w331 w334 w337]
              tunnel: [w330 w333 w336] -> w325
              tunnel: [_ _ w335] -> w322
              frame "Remove" {
                n182 = call "Remove Line.vi"("Active Line Name"=w332, "Objects"=w331) -> ("error out"=w330:errorcluster)  [unwired: 9 in]
              }
              frame "Add" {
                n183 = call "Add New Line.vi"("objects"=w334) -> ("error out"=w333:errorcluster)  [unwired: 8 in, 2 out]
              }
              frame "Edit", Default {
                n184 = call "Edit Line.vi"("Line Name"=w338, "References"=w337) -> ("error out"=w336:errorcluster, "change?"=w335:bool)  [unwired: 8 in]
              }
            }
            n185 = call "Node Change Event.vi"("error in (no error)"=w325, "Send (T)"=w322, "objects"=w324, "References in"=w323) -> ("error out"=w328:errorcluster)  [unwired: 7 in]
            n186 = call "RefreshUI Event.vi"("error in (no error)"=w328, "References in"=w323) -> ("error out"=w327:errorcluster)  [unwired: 8 in, 1 out]
          }
          event "Table": Value Change {
            # "Disable these when nothing in the table is selected."
            n187 = event-data() -> ("NewVal"=w344:i32)  [unwired: 1 in]
            n188 = Equal?(x=w344, y=-1) -> (x = y?=w342:bool)
            n189 = Select(t=T23."Disabled and Grayed Out" ("Disabled"), s=w342, f=T23."Enabled") -> (s? t:f=w340:T23)
            n190 = property on="Remove Button" class="Bool"("DisabledEnum"=w340) -> ()  [unwired: 2 in, 2 out]
            n191 = property on="Settings" class="Bool"("DisabledEnum"=w340) -> ()  [unwired: 2 in, 2 out]
          }
        }
        n192 = call "Local Error Handler.vi"("error in"=w45, "Stop in"=w47) -> ("error out"=w46:errorcluster, "Stop out"=w48:bool)  [unwired: 8 in]
      }
      n193 = call-dynamic "Event Handler.vi"("Listbox in"=w37) -> ("error out"=w36:errorcluster)  [unwired: 9 in, 1 out]
      n194 = Merge Errors(w35, w36) -> (w34:errorcluster)
    }
    frame Error {
    }
  }
  n195 = Unregister For Events(event registration refnum=w32, error in=w31) -> (error out=w30:errorcluster)
  n196 = call <vilib>:"Simple Error Handler.vi"("error in (no error)"=w30) -> ()  [unwired: 4 in, 5 out]
